vi "NewBMP280Sensor.vi"(8 "error in":errorcluster, 10 "I2C Slave Addr (0x77)":u8=119 format="%.0x", 11 "LINX I2C":refnum<class "LINX I2C.lvclass">) -> (0 "error out":errorcluster, 3 "BMP208 out":refnum<class "BMP208.lvclass">)   [LabVIEW 2020, in "BMP208.lvclass"]
uses:
  BMP208.lvclass
  LINX I2C/LINX I2C.lvclass
  Controls/td_enum_powermode.ctl
  Controls/td_enum_osrsX.ctl
panel:
  out "ChipID":u8 format="%02x"
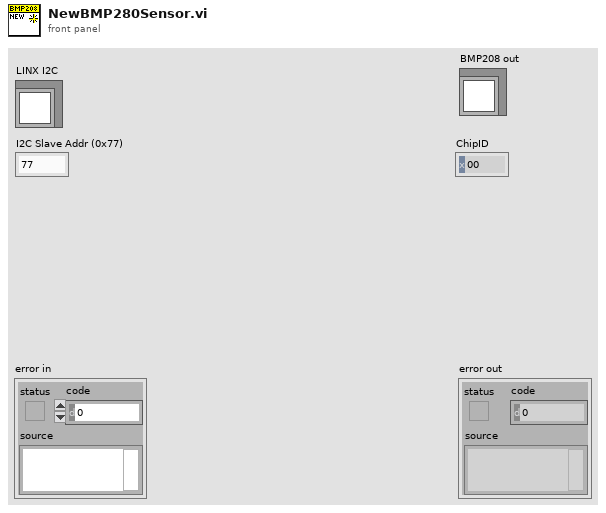
[diagram p1: front panel]
types:
  T1 = typedef "BMP208.lvclass/td_enum_osrsX.ctl" = enum16{"Skipped", "16b", "17b", "18b", "19b", "20b", "20b_2", "20b_3"}
  T2 = typedef "BMP208.lvclass/td_enum_powermode.ctl" = enum16{"Sleep", "Forced", "Forced_", "Normal"}
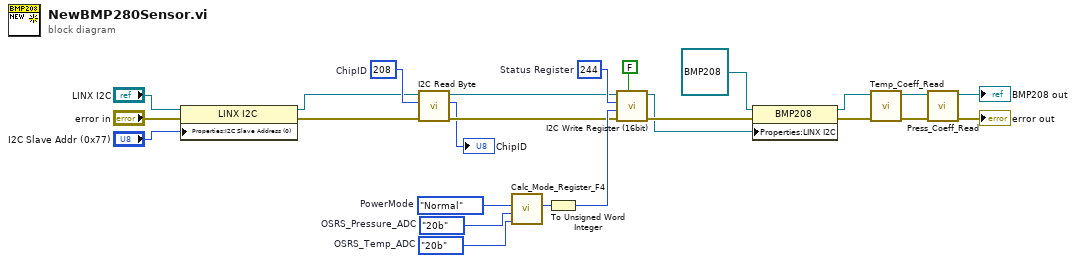
[diagram p0: block diagram]
diagram:
  w20 = u8 208  # ChipID
  w13 = td_enum_osrsX."20b"  # OSRS_Pressure_ADC
  w14 = td_enum_osrsX."20b"  # OSRS_Temp_ADC
  w12 = td_enum_powermode."Normal"  # PowerMode
  w22 = u8 244  # Status Register
  n1 = property class="LINX I2C"(reference="LINX I2C", error in="error in", "Properties:I2C Slave Address (0)"="I2C Slave Addr (0x77)") -> (reference out=w19:refnum<class "LINX I2C.lvclass">, error out=w17:errorcluster)
  n2 = call-dynamic "I2C Read Byte.vi"("error in (no error)"=w17, "Register Address"=w20, "LINX I2C in"=w19) -> ("error out"=w16:errorcluster, "Byte Read"=→"ChipID":u8, "LINX I2C out"=w18:refnum<class "LINX I2C.lvclass">)  [unwired: 6 in]
  n3 = call "Calc_Mode_Register_F4.vi"("OSRS_Temp"=w14, "OSRS_Press"=w13, "PowerMode"=w12) -> ("F4_Register"=w11:u8)  [unwired: 8 in]
  n4 = To Unsigned Word Integer(number=w11) -> (unsigned 16bit integer=w21:u16)
  n5 = call "I2C Write Register (16bit).vi"("MSB(yte) First? (F=Lo->Hi)"=FALSE, "error in (no error)"=w16, "Value"=w21, "Register Address"=w22, "LINX I2C in"=w18) -> ("error out"=w9:errorcluster, "LINX I2C out"=w6:refnum<class "LINX I2C.lvclass">)  [unwired: 5 in]
  n6 = property class="BMP208"(reference=refnum<class "BMP208.lvclass"> refnum ("BMP208 out"), error in=w9, "Properties:LINX I2C"=w6) -> (reference out=w4:refnum<class "BMP208.lvclass">, error out=w8:errorcluster)
  n7 = call "Temp_Coeff_Read.vi"("error in (no error)"=w8, "BMP208 in"=w4) -> ("error out"=w5:errorcluster, "BMP208 out"=w2:refnum<class "BMP208.lvclass">)  [unwired: 8 in]
  n8 = call "Press_Coeff_Read.vi"("error in (no error)"=w5, "BMP208 in"=w2) -> ("error out"=→"error out":errorcluster, "BMP208 out"=→"BMP208 out":refnum<class "BMP208.lvclass">)  [unwired: 8 in]
